vi "Actor Core.vi"(8 "error in":errorcluster, 11 "Simulated Wash Display Console Actor in":refnum<class "Simulated Wash Display Console Actor.lvclass">) -> (0 "error out":errorcluster, 3 "Actor out":refnum<class "Actor.lvclass">)   [LabVIEW 2019, in "Simulated Wash Display Console Actor.lvlib" / "Simulated Wash Display Console Actor.lvclass"]
doc: "(<B>Filename</B>: Actor Framework.lvlib:Actor.lvclass:Actor Core.vi)\n\nReceives messages to the actor, reacts to them, and initiates any error handling that may shut the actor down.\n\nDescendant classes may override this VI to append parallel tasks for the actor to complete while it handles messages. Overrides use the Call Parent Method node."
uses:
  Simulated Wash Display Console Actor.lvclass
  <vilib>/ActorFramework/Stop Msg/Stop Msg.lvclass
  <vilib>/ActorFramework/Actor/Actor.lvclass
  Car Wash Controller Actor/Car Wash Controller Actor Messages/Execute last step Msg/Execute last step Msg.lvclass
  C:/Workspace/CLA/Carwasher AF/Abstract Washer Display Console Actor/Abstract Washer Display Console Actor/Washer Display Console Actor.lvclass
  C:/Program Files (x86)/National Instruments/LabVIEW 2019/vi.lib/ActorFramework/Actor/Actor.lvclass
  Car Wash Controller Actor/Car Wash Controller Actor Messages/Set Vehicle Position from wash step Msg/Set Vehicle Position from wash step Msg.lvclass
  Abstract Washer Display Console Actor/Abstract Washer Display Console Actor/Washer Display Console Actor.lvclass
  Sim Entry Console Actor/Sim Entry Console Actor/Wash steps selection -Buttons.ctl
  Sim Entry Console Actor/Sim Entry Console Actor/Simulated Entry Console Actor.lvclass
panel:
  out "Time Remaining":dbl format="%.2f"
  out "Vehicle Out of Position":bool
  out "Car Wash Indicators":T1
  out "Wash Entry":string
  # "UI1"
  # "Wash Display Console"
  # "UI3."
  # "UI3A."
  # "UI3B."
  # "UI3C."
  # "UI3D."
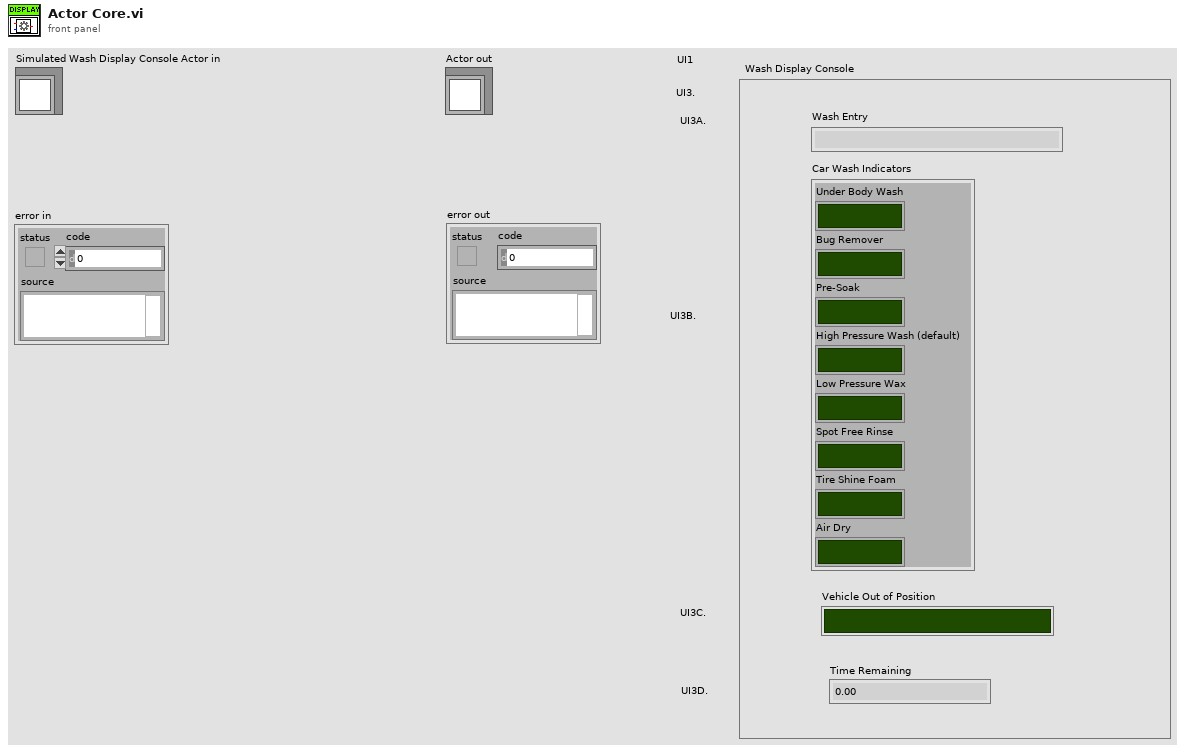
[diagram p1: front panel]
types:
  T1 = typedef "Simulated Entry Console Actor.lvlib/Simulated Entry Console Actor.lvclass/Wash steps selection -Buttons.ctl" = cluster{"Under Body Wash":bool, "Bug Remover":bool, "Pre-Soak":bool, "High Pressure Wash (default)":bool, "Low Pressure Wax":bool, "Spot Free Rinse":bool, "Tire Shine Foam":bool, "Air Dry":bool}
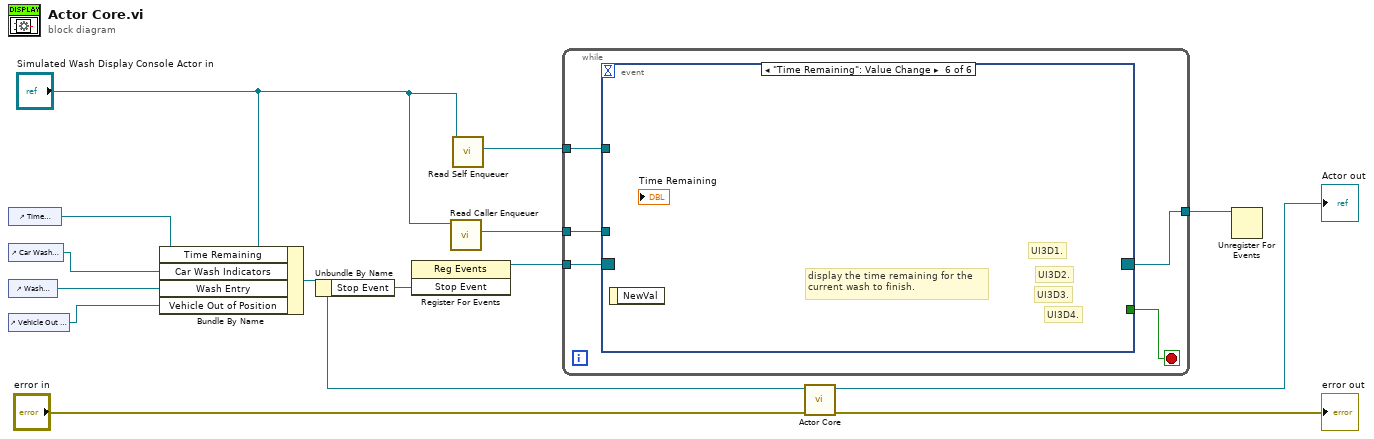
[diagram p0: block diagram]
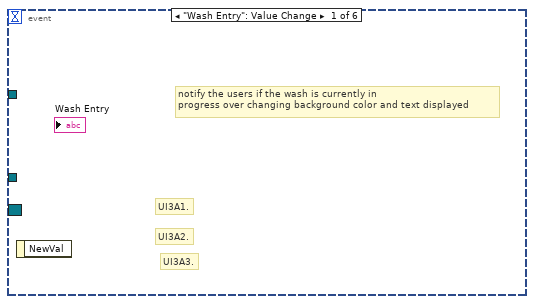
[diagram p2: hidden frame]
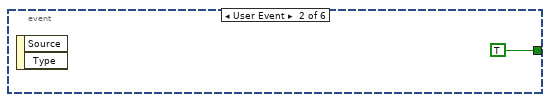
[diagram p3: hidden frame]
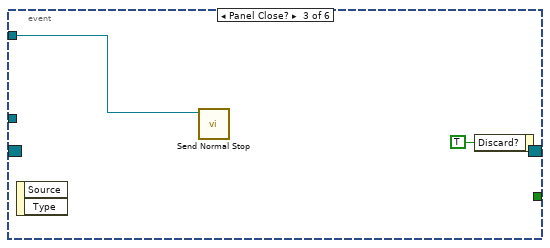
[diagram p4: hidden frame]
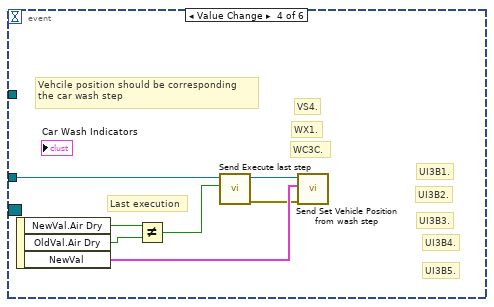
[diagram p5: hidden frame]
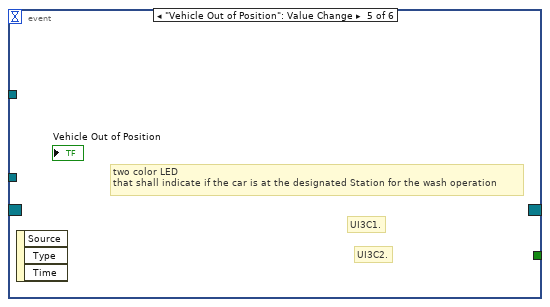
[diagram p6: hidden frame]
diagram:
  n1 = control-ref of="Time Remaining"() -> (w11:refnum<vi>)
  n2 = control-ref of="Car Wash Indicators"() -> (w10:refnum<vi>)
  n3 = control-ref of="Wash Entry"() -> (w9:refnum<vi>)
  n4 = control-ref of="Vehicle Out of Position"() -> (w8:refnum<vi>)
  n5 = Bundle By Name(cluster="Simulated Wash Display Console Actor in", "Time Remaining"=w11, "Car Wash Indicators"=w10, "Wash Entry"=w9, "Vehicle Out of Position"=w8) -> (w7:refnum<class "Simulated Wash Display Console Actor.lvclass">)
  n6 = Unbundle By Name(w7) -> ("Stop Event"=w6:refnum<user-event>)
  n7 = register-events(w6) -> (reference out=w5:refnum<event-registration>)  [unwired: 2 in, 1 out]
  n8 = call <vilib>:"Read Caller Enqueuer.vi"("Actor"="Simulated Wash Display Console Actor in") -> ("Caller Enqueuer"=w1:refnum<class "Message Enqueuer.lvclass">)  [unwired: 10 in]
  n9 = call <vilib>:"Read Self Enqueuer.vi"("Actor"="Simulated Wash Display Console Actor in") -> ("Self Enqueuer"=w3:refnum<class "Message Enqueuer.lvclass">)  [unwired: 10 in]
  n10 = while {
    tunnel: w5 -> [w19]
    tunnel: [w18] -> w4
    tunnel: w3 -> [w16]
    tunnel: w1 -> [w15]
    stop <- w17 stop-if-true
    n11 = event shown="[5] \"Time Remaining\": Value Change" {
      selector: w19 -> [_ _ _ _ _ _]
      dyn-events: [_ _ _ _ _ _] -> w18
      timeout: _ -> [_ _ _ _ _ _]
      tunnel: [_ TRUE _ _ _ _] -> w17
      tunnel: w16 -> [_ _ w21 _ _ _]
      tunnel: w15 -> [_ _ _ w26 _ _]
      event "Wash Entry": Value Change {
        # "notify the users if the wash is currently in\nprogress over changing background color and text displayed"
        # "UI3A3."
        # "UI3A2."
        # "UI3A1."
        n12 = event-data() -> ()  [unwired: 1 in, 1 out]
      }
      event User Event {
        n13 = event-data() -> ()  [unwired: 1 in, 2 out]
      }
      event Panel Close? {
        n14 = event-data() -> ()  [unwired: 1 in, 2 out]
        n15 = call <vilib>:"Send Normal Stop.vi"("Message Enqueuer"=w21) -> ()  [unwired: 10 in, 1 out]
        n16 = event-data("Discard?"=TRUE) -> ()  [unwired: 1 in, 1 out]
      }
      event Value Change {
        # "Vehcile position should be corresponding\nthe car wash step"
        # "WC3C."
        # "WX1."
        # "VS4."
        # "Last execution"
        # "UI3B5."
        # "UI3B4."
        # "UI3B3."
        # "UI3B2."
        # "UI3B1."
        n17 = event-data() -> ("NewVal.Air Dry"=w29:bool, "OldVal.Air Dry"=w28:bool, "NewVal"=w24:T1)  [unwired: 1 in]
        n18 = Not Equal?(x=w29, y=w28) -> (x != y?=w27:bool)
        n19 = call "Send Execute last step.vi"("Last Step done"=w27, "Message Enqueuer"=w26) -> ("error out"=w23:errorcluster, "Message Enqueuer out"=w25:refnum<class "Message Enqueuer.lvclass">)  [unwired: 8 in]
        n20 = call "Send Set Vehicle Position from wash step.vi"("error in (no error)"=w23, "Car Wash Steps"=w24, "Message Enqueuer"=w25) -> ()  [unwired: 7 in, 2 out]
      }
      event "Vehicle Out of Position": Value Change {
        # "two color LED\nthat shall indicate if the car is at the designated Station for the wash operation"
        # "UI3C2."
        # "UI3C1."
        n21 = event-data() -> ()  [unwired: 1 in, 3 out]
      }
      event "Time Remaining": Value Change {
        # "display the time remaining for the\ncurrent wash to finish."
        # "UI3D4."
        # "UI3D3."
        # "UI3D2."
        # "UI3D1."
        n22 = event-data() -> ()  [unwired: 1 in, 1 out]
      }
    }
  }
  n23 = call-parent "Actor Core.vi"("error in"="error in", "Actor in"=w7) -> ("error out"=→"error out":errorcluster, "Actor out"=→"Actor out":refnum<class "Actor.lvclass">)  [unwired: 8 in]
  n24 = Unregister For Events(event registration refnum=w4) -> ()  [unwired: 1 in, 1 out]
